vi "Publish MPReading.vi"(8 "error in (no error)":errorcluster, 11 "CS++DMM in":refnum<class "CS++DMM.lvclass">) -> (0 "error out":errorcluster, 3 "CS++DMM out":refnum<class "CS++DMM.lvclass">)   [LabVIEW 2013, in "CS++DMM.lvlib" / "CS++DMM.lvclass"]
doc: "Publish Multi-Point Reading to PV."
uses:
  CS++DMM.lvclass
  Core/Classes/CS++ProcessVariables/ProcessVariable/PV.lvclass
  CS++DMM.lvclass/CS++DMM.ctl
  Core/Classes/CS++ProcessVariables/PVConnection/PVConnection.lvclass
  Core/Classes/CS++ProcessVariables/ProcessVariable/PV.lvclass/PV.ctl
  Core/Classes/CS++ProcessVariables/ProcessVariable/Write Data.vi
  Core/Classes/CS++ProcessVariables/ProcessVariable/Write Timestamp.vi
  Core/Classes/CS++ProcessVariables/ProcessVariable/Write Quality.vi
  Core/Classes/CS++ProcessVariables/ProcessVariable/Write status.vi
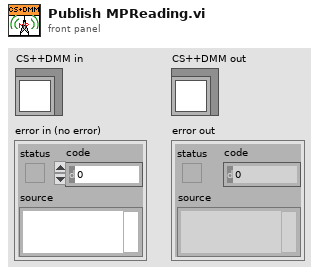
[diagram p1: front panel]
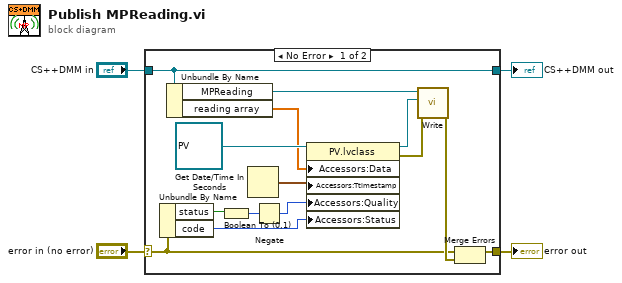
[diagram p0: block diagram]
diagram:
  n1 = case shown="No Error" "error in (no error)" {
    selector: "error in (no error)" -> [w6 w20]
    tunnel: [w5 w20] -> w3
    tunnel: [w9 w19] -> w1
    tunnel: "CS++DMM in" -> [w9 w19]
    frame No Error {
      n2 = Unbundle By Name(w6) -> ("status"=w14:bool, "code"=w11:i32)
      n3 = Unbundle By Name(w9) -> ("MPReading"=w18:refnum<class "PVConnection.lvclass">, "reading array"=w16:dbl[])
      n4 = Boolean To (0,1)(Boolean=w14) -> (0, 1=w13:i16)
      n5 = Get Date/Time In Seconds() -> (seconds since 1Jan1904=w15:timestamp)
      n6 = Negate(x=w13) -> (-x=w12:i16)
      n7 = property class="PV.lvclass"(reference=refnum<class "PV.lvclass"> refnum ("CS++ProcessVariables.lvlib:PV.lvclass"), "Accessors:Data"=w16, "Accessors:Ttimestamp"=w15, "Accessors:Quality"=w12, "Accessors:Status"=w11) -> (reference out=w10:refnum<class "PV.lvclass">, error out=w7:errorcluster)  [unwired: 1 in]
      n8 = call-dynamic "Write.vi"("error in (no error)"=w7, "PV"=w10, "PVConnection in"=w18) -> ("error out"=w8:errorcluster)  [unwired: 7 in, 1 out]
      n9 = Merge Errors(w6, w8) -> (w5:errorcluster)
    }
    frame Error {
    }
  }
  "error out" <- w3
  "CS++DMM out" <- w1
